vi "cvt version constant.vi"() -> (3 "current version":string="1.0.0.0")   [LabVIEW 2013, in "CVT configuration.lvclass"]
uses:
  CVT configuration.lvclass
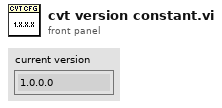
[diagram p1: front panel]
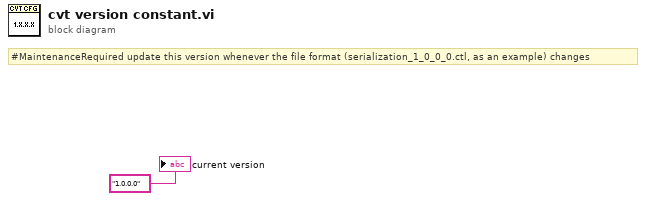
[diagram p0: block diagram]
diagram:
  # "#MaintenanceRequired update this version whenever the file format (serialization_1_0_0_0.ctl, as an example) changes"
  "current version" <- "1.0.0.0" ("current version")
